vi "read_temps(SubVI).vi"(11 "VISA Refnum in":refnum<visa-resource-name>) -> (3 "Array":dbl[](array[numeric]))   [LabVIEW 2013]
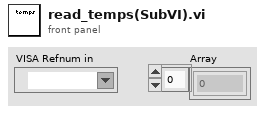
[diagram p1: front panel]
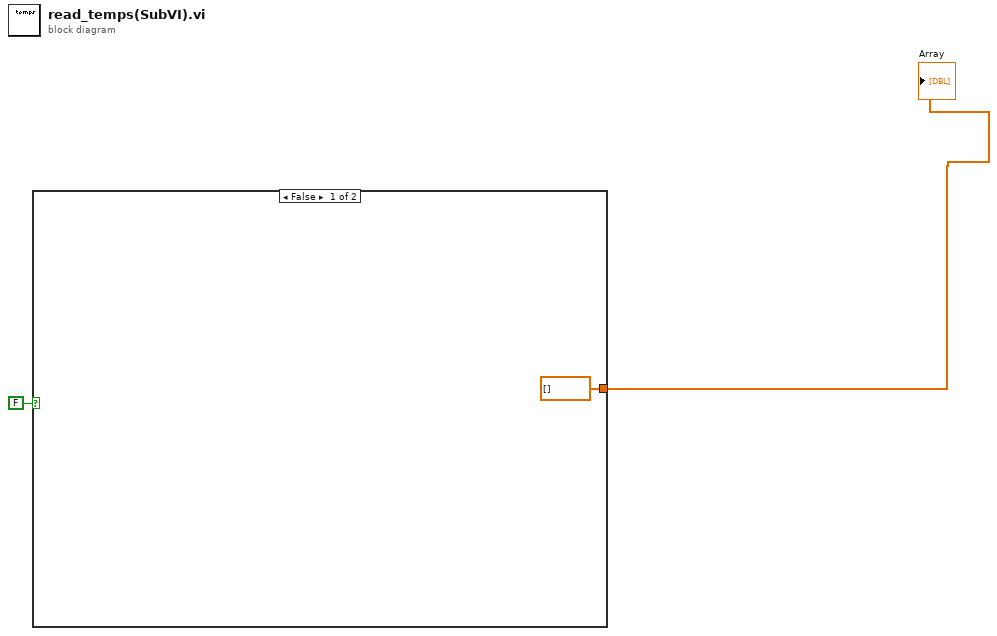
[diagram p0: block diagram]
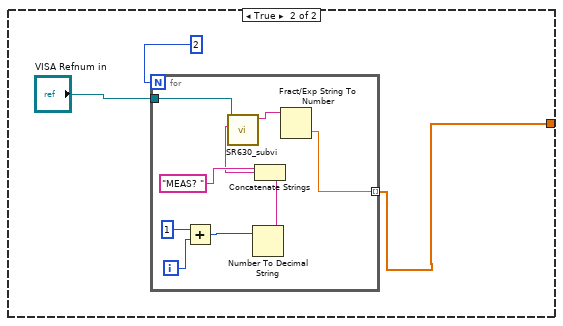
[diagram p2: hidden frame]
diagram:
  n1 = case shown="False" FALSE {
    tunnel: [dbl[] [] w6] -> w2
    frame False {
    }
    frame True {
      n2 = for {
        N: 2 ("dimension size") -> [_]
        tunnel: "VISA Refnum in" -> [w15]
        tunnel: [w13] -> w6 mode=indexing
        i -> [w12]
        n3 = Add(x=1, y=w12) -> (x+y=w10:i32)
        n4 = Number To Decimal String(number=w10) -> (decimal integer string=w9:string)  [unwired: 1 in]
        n5 = Concatenate Strings("MEAS? " ("Write Buffer"), w9) -> (w7:string)
        n6 = call "SR630_subvi.vi"("Write Buffer"=w7, "VISA Refnum in"=w15) -> ("read buffer"=w14:string)  [unwired: 9 in]
        n7 = Fract/Exp String To Number(string=w14) -> (number=w13:dbl)  [unwired: 3 in, 1 out]
      }
    }
  }
  "Array" <- w2
